vi "PIM Initialize Test.vi"(0 "PIM Test Parameters":T2={"Stimulus"={"C1 Pwr dBm"=0.0, "C2 Pwr dBm"=0.0, "Power Units"=enum."dBm", "Meas Type"=enum."Time", "C1 Freq MHz"=0.0, "C2 Freq MHz"=0.0, "Swept Freq Step"=0}, "Measure"={"IM Order"=0, "Direction"=0, "Averaging"=1, "ALC ON?"=TRUE, "Peak Hold?"=TRUE, "Peak last N"=1, "Ref Level dBm"=-100.0, "Ref Units"=enum."dBm", "Num Samples"=1, "Sample units"=enum."Sample(s)", "Update Rate (s)"=0.0, "DUT PORT"=enum."Port 1", "Percent (%)"=100}, "Display"={"Power Scale"={"yRange_min"=0, "yRange_max"=0}, "xRange_span"=5}} {"Stimulus"."Swept Freq Step" items=[".2", ".4", "1.0", "2.0"]; "Measure"."Averaging" items=["None", "Minimum", "Normal", "High", "Maximum"]; "Measure"."Direction" items=["Reverse", "Forward", "Auxiliary"]; "Measure"."IM Order" items=["3rd", "5th", "7th", "9th", "11th", "13th", "15th", "17th", "19th", "21st", "23rd", "25th", "27th", "29th", "31st", "33rd"]}, 1 "PIM Instrument":T13, 11 "error in (no error)":errorcluster, 12 "Seq Count":u32, 13 "Driver Ref in":T1) -> (2 "Instrument In-Cal?":bool, 3 "TestSetDef":T12={"General"={"ID"=0, "Model"="", "Dual Port?"=FALSE, "Options"="", "Options"={"E"=FALSE, "K"=FALSE, "H"=FALSE, "W"=FALSE, "F"=FALSE}, "Cal File"=path ""}, "Receiver"={"Fstart, MHz"=0.0, "Fstop MHz"=0.0, "Fstep MHz"=0.0, "IF, MHz"=0.0}, "RX Band"={"Fstart, MHz"=0.0, "Fstop MHz"=0.0}, "TX 1"={"Fstart, MHz"=0.0, "Fstop MHz"=0.0, "Pmax, dBm"=0.0, "Pstep, dB"=0.0}, "TX 2"={"Fstart, MHz"=0.0, "Fstop MHz"=0.0, "Pmax, dBm"=0.0, "Pstep, dB"=0.0}, "Low-side?"=TRUE}, 4 "TestSet Model":string, 6 "Serial Number":string, 8 "Corrected Test Params":T2={"Stimulus"={"C1 Pwr dBm"=0.0, "C2 Pwr dBm"=0.0, "Power Units"=enum."dBm", "Meas Type"=enum."Time", "C1 Freq MHz"=0.0, "C2 Freq MHz"=0.0, "Swept Freq Step"=0}, "Measure"={"IM Order"=0, "Direction"=0, "Averaging"=1, "ALC ON?"=TRUE, "Peak Hold?"=TRUE, "Peak last N"=1, "Ref Level dBm"=-100.0, "Ref Units"=enum."dBm", "Num Samples"=1, "Sample units"=enum."Sample(s)", "Update Rate (s)"=0.0, "DUT PORT"=enum."Port 1", "Percent (%)"=100}, "Display"={"Power Scale"={"yRange_min"=0, "yRange_max"=0}, "xRange_span"=5}} {"Stimulus"."Swept Freq Step" items=[".2", ".4", "1.0", "2.0"]; "Measure"."Averaging" items=["None", "Minimum", "Normal", "High", "Maximum"]; "Measure"."Direction" items=["Reverse", "Forward", "Auxiliary"]; "Measure"."IM Order" items=["3rd", "5th", "7th", "9th", "11th", "13th", "15th", "17th", "19th", "21st", "23rd", "25th", "27th", "29th", "31st", "33rd"]}, 14 "Driver Ref out":T1, 15 "error out":errorcluster)   [LabVIEW 2011]
uses:
  TypeDefs/PIM Test Parameters.ctl
  TypeDefs/PIM Stimulus Parameters.ctl
  BPIMCore/HW IO/PIM Sweep Step Size.ctl
  TypeDefs/PIM Measurement Parameters.ctl
  BPIMCore/HW IO/IMOrder.ctl
  BPIMCore/HW IO/MeasMode.ctl
  BPIMCore/HW IO/HW Averaging.ctl
  TypeDefs/PIM Meas Units.ctl
  BPIMCore/HW IO/DUTport.ctl
  TypeDefs/PIM Display Parameters.ctl
  typedefs/Instrument Record.ctl
  drivers/PIM/PIM Driver Ref.ctl
  BPIMCore/HW IO/Test Set Definition.ctl
  drivers/PIM/PIM Command.ctl
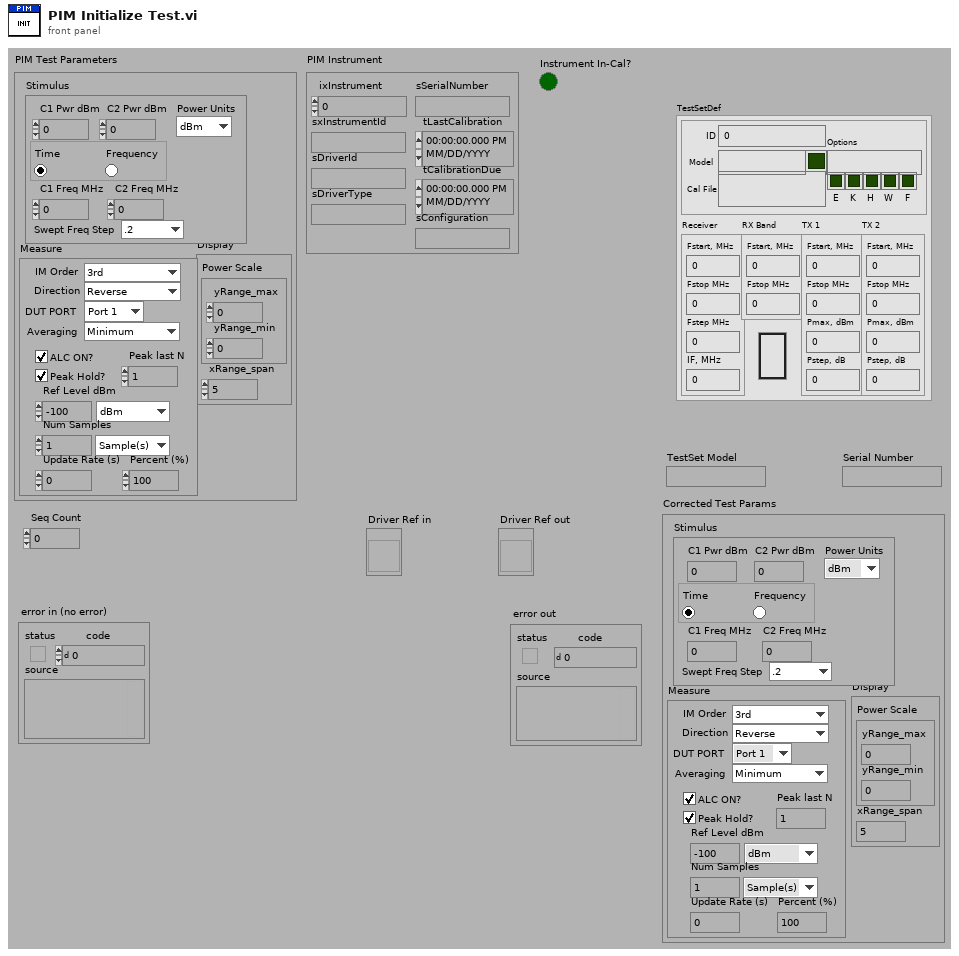
[diagram p1: front panel]
types:
  T1 = typedef "PIM Driver Ref.ctl" = refnum<vi>
  T2 = typedef "PIM Test Parameters.ctl" = cluster{"Stimulus":T3, "Measure":T5, "Display":T11}
  T3 = typedef "PIM Stimulus Parameters.ctl" = cluster{"C1 Pwr dBm":dbl, "C2 Pwr dBm":dbl, "Power Units":enum16{"dBm", "Watts"}, "Meas Type":enum32{"Time", "Frequency"}, "C1 Freq MHz":dbl, "C2 Freq MHz":dbl, "Swept Freq Step":T4}
  T4 = typedef "PIM Sweep Step Size.ctl" = u16
  T5 = typedef "PIM Measurement Parameters.ctl" = cluster{"IM Order":T6, "Direction":T7, "Averaging":T8, "ALC ON?":bool, "Peak Hold?":bool, "Peak last N":u32, "Ref Level dBm":dbl, "Ref Units":enum16{"dBm", "dBc"}, "Num Samples":u32, "Sample units":T9, "Update Rate (s)":dbl, "DUT PORT":T10, "Percent (%)":u8}
  T6 = typedef "IMOrder.ctl" = u8
  T7 = typedef "MeasMode.ctl" = u16
  T8 = typedef "HW Averaging.ctl" = u16
  T9 = typedef "PIM Meas Units.ctl" = enum16{"Sample(s)", "Second(s)", "Sweep(s)"}
  T10 = typedef "DUTport.ctl" = enum16{"Port 1", "Port 2"}
  T11 = typedef "PIM Display Parameters.ctl" = cluster{"Power Scale":cluster{"yRange_min":i32, "yRange_max":i32}, "xRange_span":u32}
  T12 = typedef "Test Set Definition.ctl" = cluster{"General":cluster{"ID":u32, "Model":string, "Dual Port?":bool, "Options":string, "Options":cluster{"E":bool, "K":bool, "H":bool, "W":bool, "F":bool}, "Cal File":path}, "Receiver":cluster{"Fstart, MHz":dbl, "Fstop MHz":dbl, "Fstep MHz":dbl, "IF, MHz":dbl}, "RX Band":cluster{"Fstart, MHz":dbl, "Fstop MHz":dbl}, "TX 1":cluster{"Fstart, MHz":dbl, "Fstop MHz":dbl, "Pmax, dBm":dbl, "Pstep, dB":dbl}, "TX 2":cluster{"Fstart, MHz":dbl, "Fstop MHz":dbl, "Pmax, dBm":dbl, "Pstep, dB":dbl}, "Low-side?":bool}
  T13 = typedef "Instrument Record.ctl" = cluster{"ixInstrument":i32, "sxInstrumentId":string, "sDriverId":string, "sDriverType":string, "sSerialNumber":string, "tLastCalibration":timestamp, "tCalibrationDue":timestamp, "sConfiguration":string}
  T14 = typedef "PIM Command.ctl" = enum16{"LOAD", "KEEP ALIVE", "VALIDATE", "INITIALIZE", "PRESET", "GET CALIBRATION", "SET STIMULUS", "TOGGLE TX POWER", "SET TX ON", "SET TX OFF", "MEASURE", "UNLOAD"}
  T15 = typedef "PIM Stimulus.ctl" = cluster{"Carrier Frequencies":cluster{"C1 Freq, MHz":dbl, "C2 Freq, MHz":dbl}, "Carrier Powers":cluster{"C1 Power,dBm":dbl, "C2 Power, dBm":dbl}, "Measurement Parameters":T16, "Measurement Setup":cluster{"Meas Type":enum32{"Time", "Frequency"}, "TXStep":T4}}
  T16 = typedef "PIM Cmd Params.ctl" = cluster{"IM Order":T6, "Averaging":T8, "Direction":T7, "Enable ALC?":bool, "Enable SingleIM?":bool, "Display Units":T17, "VA Hold?":bool, "DUT PORT":T10}
  T17 = typedef "display_unit_format.ctl" = enum16{"dBm", "dBc"}
  T18 = typedef "LVDateTimeRec.ctl" = cluster{"fractional second":dbl, "second":i32, "minute":i32, "hour":i32, "day of month":i32, "month":i32, "year":i32, "day of week":i32, "day of year":i32, "DST":i32}
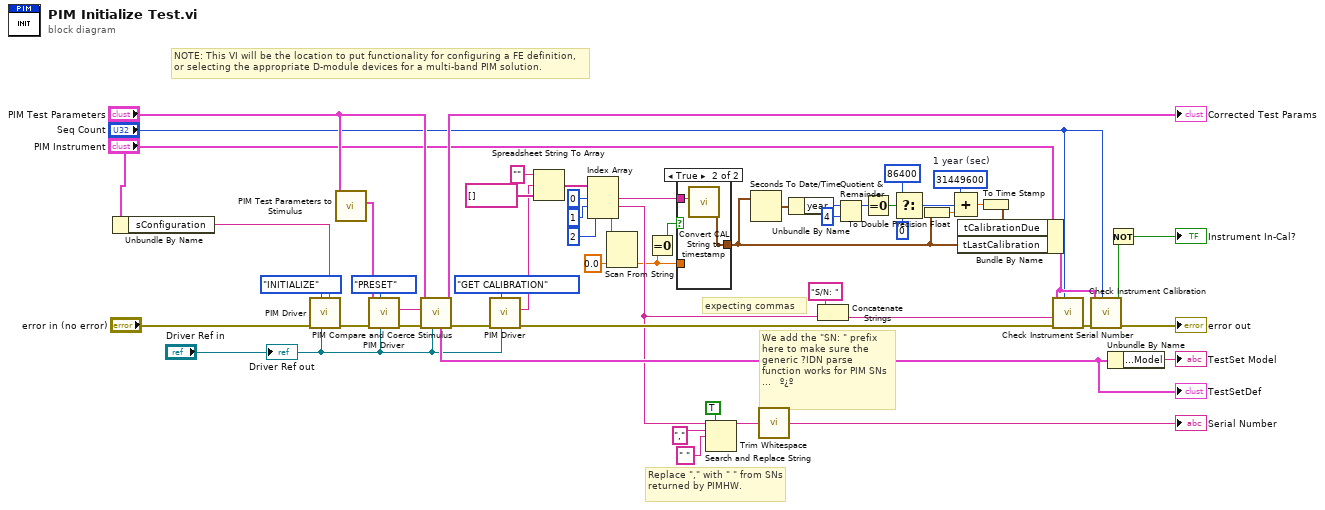
[diagram p0: block diagram]
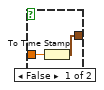
[diagram p2: hidden frame]
diagram:
  w16 = 31449600  # 1 year (sec)
  # "expecting commas"
  # "Replace \",\" with \" \" from SNs returned by PIMHW."
  # "NOTE: This VI will be the location to put functionality for configuring a FE definition, or selecting the appropriate D-module devices for a multi-band PIM solution."
  # "We add the \"SN: \" prefix here to make sure the generic ?IDN parse function works for PIM SNs ...   º¿º"
  n1 = Unbundle By Name("PIM Instrument") -> ("sConfiguration"=w55:string)
  n2 = call "PIM Driver.vi"("PIM Driver Name/Configuration"=w55, "Driver Ref (null)"="Driver Ref in", "PIM Command"=PIM_Command."INITIALIZE", "error in (no error)"="error in (no error)") -> ("error out"=w38:errorcluster)  [unwired: 1 in, 6 out]
  n3 = call "PIM Test Parameters to Stimulus.vi"("PIM Test Parameters"="PIM Test Parameters") -> ("PIM Measurement Stimulus"=w32:T15)  [unwired: 10 out]
  n4 = call "PIM Driver.vi"("Driver Ref (null)"="Driver Ref in", "PIM Command"=PIM_Command."PRESET", "error in (no error)"=w38, "Stimulus"=w32) -> ("error out"=w41:errorcluster, "Variant Output"=w43:string)  [unwired: 1 in, 5 out]
  n5 = call "PIM Compare and Coerce Stimulus.vi"("Driver Ref (null)"="Driver Ref in", "error in (no error)"=w41, "Flat TestSetDef Params"=w43, "PIM Test Parameters"="PIM Test Parameters") -> ("error out"=w37:errorcluster, "Corrected Test Params"=→"Corrected Test Params":T2, "TestSetDef"=w42:T12)  [unwired: 5 out]
  "TestSetDef" <- w42
  n6 = call "PIM Driver.vi"("Driver Ref (null)"="Driver Ref in", "PIM Command"=PIM_Command."GET CALIBRATION", "error in (no error)"=w37) -> ("error out"=w34:errorcluster, "Variant Output"=w35:string)  [unwired: 2 in, 5 out]
  n7 = Spreadsheet String To Array(format string="", spreadsheet string=w35, array type (2D Dbl)=string[] []) -> (array=w54:string[])  [unwired: 1 out]
  n8 = Index Array(array=w54, index #1=0 ("index"), index #2=1 ("index"), index #3=2 ("index")) -> (element #1=w50:string, element #2=w23:string, element #3=w5:string)
  n9 = Scan From String(input string=w5, default 1=0.0 ("default value 1")) -> (output 1=w3:dbl)  [unwired: 3 in, 3 out]
  n10 = Equal To 0?(x=w3) -> (x = 0?=w2:bool)
  n11 = case shown="True" w2 {
    tunnel: w50 -> [_ w60]
    tunnel: w3 -> [w58 _]
    tunnel: [w57 w59] -> w1
    frame False {
      n12 = To Time Stamp(1:w58) -> (0:w57:timestamp)
    }
    frame True {
      n13 = call "Convert CAL String to timestamp.vi"("abbreviated date string"=w60) -> ("time stamp"=w59:timestamp)  [unwired: 10 out]
    }
  }
  n14 = Search and Replace String(replace all?=TRUE ("replace all? (F)"), input string=w23, search string="," ("delimiter (Tab)"), replace string=" " ("replace string (\"\")")) -> (result string=w25:string)  [unwired: 1 in, 6 out]
  n15 = Seconds To Date/Time(time stamp (now)=w1) -> (date time rec=w20:T18)  [unwired: 1 in]
  n16 = call <vilib>:"Trim Whitespace.vi"("string"=w25) -> ("trimmed string"=→"Serial Number":string)  [unwired: 1 in]
  n17 = Unbundle By Name(w20) -> ("year"=w19:i32)
  n18 = Concatenate Strings("S/N: ", w23) -> (w46:string)
  n19 = Quotient & Remainder(x=w19, y=4) -> (x-y*floor(x/y)=w17:i32)  [unwired: 1 out]
  n20 = Equal To 0?(x=w17) -> (x = 0?=w15:bool)
  n21 = Select(t=86400 ("y"), s=w15, f=0 ("y")) -> (s? t:f=w12:i32)
  n22 = To Double Precision Float(number=w1) -> (double precision float=w10:dbl)
  n23 = Compound Arithmetic op=ADD(w16, w12, w10) -> (w11:dbl)
  n24 = To Time Stamp(1:w11) -> (0:w9:timestamp)
  n25 = Bundle By Name(cluster="PIM Instrument", "tCalibrationDue"=w9, "tLastCalibration"=w1) -> (w48:T13)
  n26 = call "Check Instrument Serial Number.vi"("Seq Count"="Seq Count", "error in (no error)"=w34, "Instrument IDN String (\"\")"=w46, "Instrument Record"=w48) -> ("error out"=w49:errorcluster)  [unwired: 7 out]
  n27 = call "Check Instrument Calibration.vi"("Seq Count"="Seq Count", "error in (no error)"=w49, "Instrument Record"=w48) -> ("error out"=→"error out":errorcluster, "Cal Expired?"=w40:bool)  [unwired: 7 out]
  n28 = Not(x=w40) -> (.not. x?=→"Instrument In-Cal?":bool)
  n29 = Unbundle By Name(w42) -> ("General.Model"=→"TestSet Model":string)
  "Driver Ref out" <- "Driver Ref in"
